vi "solar_app SOLARini Read (2DSTR).vi"(4 "Delimiters (1D,2D)":string[](array[string]), 5 "Write If Not Found? (T)":bool=TRUE, 6 "Comment (Create only)":string, 7 "Section (\"\"=solar)":string, 9 "Default Value (STR)":string[][](array[string]), 10 "Key":string) -> (1 "Value (STR) out":string[][](array[string]), 2 "Found?":bool)   [LabVIEW 2018]
doc: "This reads a 2D string array configuration key from the solar.ini configuration file."
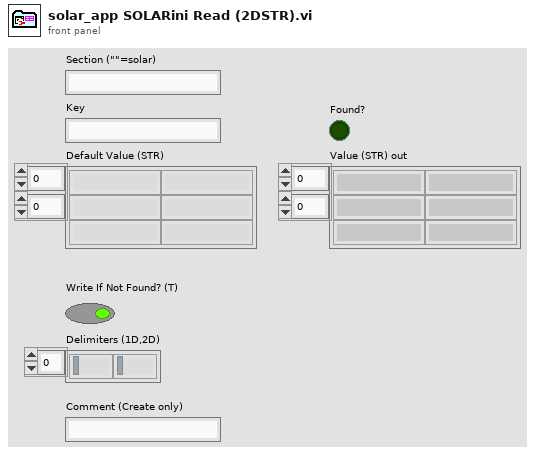
[diagram p1: front panel]
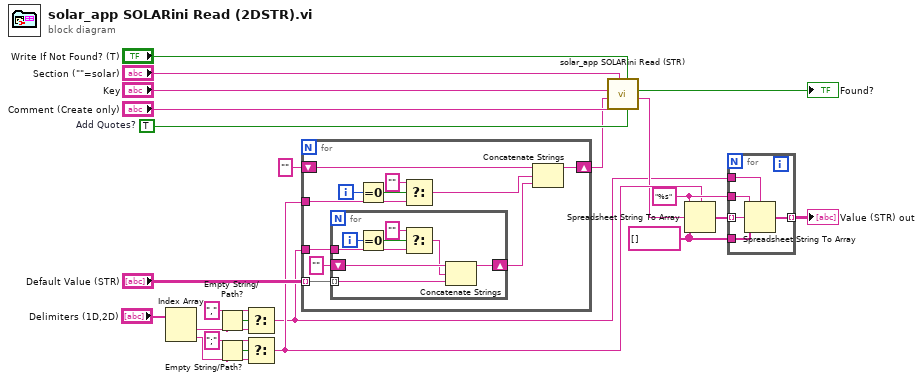
[diagram p0: block diagram]
diagram:
  w5 = string[] []
  w6 = "%s" ("format string")
  w21 = TRUE  # Add Quotes?
  n1 = Index Array(array="Delimiters (1D,2D)") -> (element #1=w16:string, element #2=w15:string)  [unwired: 2 in]
  n2 = Empty String/Path?(string/path=w16) -> (empty?=w17:bool)
  n3 = Empty String/Path?(string/path=w15) -> (empty?=w13:bool)
  n4 = Select(t=",", s=w17, f=w16) -> (s? t:f=w2:string)
  n5 = Select(t=";", s=w13, f=w15) -> (s? t:f=w4:string)
  n6 = for {
    tunnel: w2 -> [w33]
    tunnel: w4 -> [w29]
    shift-right: [w26] -> w8
    shift-left: "" -> [w25]
    tunnel: "Default Value (STR)" -> [w24] mode=indexing
    i -> [w30]
    n7 = for {
      shift-right: [w42] -> w32
      shift-left: "" -> [w41]
      tunnel: w33 -> [w38]
      tunnel: w24 -> [w35] mode=indexing
      i -> [w40]
      n8 = Equal To 0?(x=w40) -> (x = 0?=w39:bool)
      n9 = Select(t="", s=w39, f=w38) -> (s? t:f=w37:string)
      n10 = Concatenate Strings(w41, w37, w35) -> (w42:string)
    }
    n11 = Equal To 0?(x=w30) -> (x = 0?=w31:bool)
    n12 = Select(t="", s=w31, f=w29) -> (s? t:f=w27:string)
    n13 = Concatenate Strings(w25, w27, w32) -> (w26:string)
  }
  n14 = call "solar_app SOLARini Read (STR).vi"("Add Quotes? (T)"=w21, "Write If Not Found? (T)"="Write If Not Found? (T)", "Comment (Create only)"="Comment (Create only)", "Section (\"\"=solar)"="Section (\"\"=solar)", "Default Value (STR)"=w8, "Key"="Key") -> ("Value (STR) out"=w3:string, "Found?"=→"Found?":bool)  [unwired: 4 in]
  n15 = Spreadsheet String To Array(delimiter (Tab)=w4, format string=w6, spreadsheet string=w3, array type (2D Dbl)=w5) -> (array=w7:string[])
  n16 = for {
    tunnel: w7 -> [w46] mode=indexing
    tunnel: w6 -> [w45]
    tunnel: w5 -> [w47]
    tunnel: w2 -> [w44]
    tunnel: [w43] -> w1 mode=indexing
    n17 = Spreadsheet String To Array(delimiter (Tab)=w44, format string=w45, spreadsheet string=w46, array type (2D Dbl)=w47) -> (array=w43:string[])
  }
  "Value (STR) out" <- w1
